vi "VI Tree.vi"   [LabVIEW 2013, in "Watts Up Series.lvlib"]
doc: "This is the instrument driver for the <INSTRUMENT NAME>. The VI Tree displays all the user-callable VIs of the instrument driver in an organized table."
uses:
  <instrlib>/Watts Up Series/Watts Up Series.lvlib
panel:
  # "(c) 2014 <Enter Company Name Here>.  ALL RIGHTS RESERVED."
  # "SEE DIAGRAM\nFOR VI TREE."
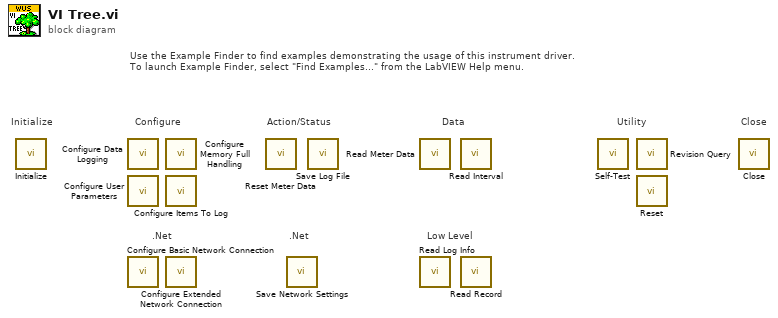
[diagram p0: block diagram]
diagram:
  # ".Net"
  # "Action/Status"
  # ".Net"
  # "Low Level"
  # "Use the Example Finder to find examples demonstrating the usage of this instrument driver.\nTo launch Example Finder, select \"Find Examples...\" from the LabVIEW Help menu."
  # "Configure"
  # "Utility"
  # "Data"
  # "Close"
  # "Initialize"
  n1 = call <instrlib>:"Initialize.vi"() -> ()  [unwired: 10 in, 2 out]
  n2 = call <instrlib>:"Configure Data Logging.vi"() -> ()  [unwired: 10 in, 2 out]
  n3 = call <instrlib>:"Configure User Parameters.vi"() -> ()  [unwired: 10 in, 2 out]
  n4 = call <instrlib>:"Configure Basic Network Connection.vi"() -> ()  [unwired: 10 in, 2 out]
  n5 = call <instrlib>:"Configure Memory Full Handling.vi"() -> ()  [unwired: 10 in, 2 out]
  n6 = call <instrlib>:"Configure Items To Log.vi"() -> ()  [unwired: 10 in, 2 out]
  n7 = call <instrlib>:"Configure Extended Network Connection.vi"() -> ()  [unwired: 10 in, 2 out]
  n8 = call <instrlib>:"Reset Meter Data.vi"() -> ()  [unwired: 10 in, 2 out]
  n9 = call <instrlib>:"Save Network Settings.vi"() -> ()  [unwired: 10 in, 2 out]
  n10 = call <instrlib>:"Save Log File.vi"() -> ()  [unwired: 10 in, 2 out]
  n11 = call <instrlib>:"Read Meter Data.vi"() -> ()  [unwired: 9 in, 3 out]
  n12 = call <instrlib>:"Read Log Info.vi"() -> ()  [unwired: 9 in, 3 out]
  n13 = call <instrlib>:"Read Interval.vi"() -> ()  [unwired: 9 in, 3 out]
  n14 = call <instrlib>:"Read Record.vi"() -> ()  [unwired: 9 in, 3 out]
  n15 = call <instrlib>:"Self-Test.vi"() -> ()  [unwired: 8 in, 4 out]
  n16 = call <instrlib>:"Revision Query.vi"() -> ()  [unwired: 8 in, 4 out]
  n17 = call <instrlib>:"Reset.vi"() -> ()  [unwired: 10 in, 2 out]
  n18 = call <instrlib>:"Close.vi"() -> ()  [unwired: 11 in, 1 out]
